vi "Write Flattened Data.vi"(8 "error in (no error)":errorcluster, 10 "Flattened Data":string, 11 "Endpoint in":refnum<class "Endpoint.lvclass">) -> (0 "error out":errorcluster, 3 "Endpoint out":refnum<class "Endpoint.lvclass">)   [LabVIEW 2020, in "Stream-Simple-Msg.lvlib" / "Endpoint.lvclass"]
uses:
  Endpoint.lvclass
  <vilib>/IlluminatedG/lv-stream/stream/Stream.lvclass/Stream.ctl
  <vilib>/IlluminatedG/lv-stream/stream/Dispatch Sniffer Data.vi
  <vilib>/IlluminatedG/lv-stream/stream/Prepared.vi
  <vilib>/IlluminatedG/lv-stream/Endpoint/Cast Sniffer Callback.vi
  <vilib>/Utility/error.llb/Error Cluster From Error Code.vi
  <vilib>/IlluminatedG/lv-stream/stream/Stream.lvclass
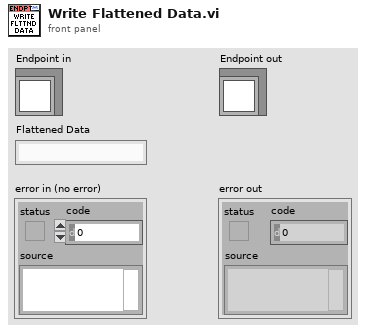
[diagram p1: front panel]
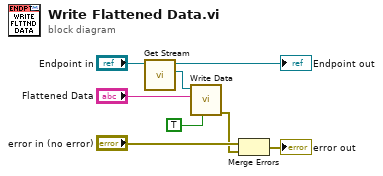
[diagram p0: block diagram]
diagram:
  n1 = call "Get Stream.vi"("Endpoint in"="Endpoint in") -> ("Stream"=w8:refnum<class "Stream.lvclass">, "Endpoint out"=→"Endpoint out":refnum<class "Endpoint.lvclass">)  [unwired: 8 in, 1 out]
  n2 = call <vilib>:"Write Data.vi"("Prepend Length? (F)"=TRUE, "Data"="Flattened Data", "Stream in"=w8) -> ("error out"=w3:errorcluster)  [unwired: 7 in, 1 out]
  n3 = Merge Errors("error in (no error)", w3) -> (→"error out":errorcluster)
